vi "Quick Format.vi"(6 "Variant in":variant, 7 "Shift Pressed?":bool, 8 "error in":errorcluster, 10 "QD Combo Box Ref":refnum<vi>, 11 "QD Launch VI Ref":refnum<vi>) -> (0 "error out":errorcluster, 4 "Variant out":variant)   [LabVIEW 2019, in "Quick Format QD.lvlib"]
doc: "Formats selected controls, indicators, and/or constants. The format descriptor must be entered in the Quick Drop window before activating this plugin.\n\nAccepted format descriptors are as follows. The descriptors are not case sensitive.\nDecimal (numeric) - d, dec\nHexadecimal (numeric, string) - h, x, hex\nOctal (numeric) - o, oct\nBinary (numeric) - b, bin\nSI (numeric) - si\nSI notation with specific units (numeric) - freq, sec, volt, amp, ohm, watt\nDecimal notation with specific units (numeric) - db, dbm, dbc\nLocal Time (numeric and timestamp) - time\nUTC Time (numeric and timestamp) - utc\nNormal Display (string) - n, norm\nSlash Codes (string) - \\, slash\nPassword Display (string) - p, pass\nCustom Code (numeric, timestamp) - any valid display format (for example: %f)\n\nAny setting that is applied to a string forces the Display Style to be visible.\nHexadecimal, Octal, and Binary settings applied to numerics forces the radix to be visible.\nHexadecimal, Octal, and Binary settings applied to numerics set the number of displayed digits based on the data type.\nAny elements inside of arrays and clusters are recursively processed.\n\nDefault Shortcut - [5]"
uses:
  Quick Format QD.lvlib
panel:
  # "THE SOFTWARE IS PROVIDED “AS IS” AND THE AUTHOR DISCLAIMS ALL WARRANTIES WITH REGARD TO THIS SOFTWARE INCLUDING ALL IMPLIED WARRANTIES OF MERCHANTABILITY AND FITNESS. IN NO EVENT SHALL THE AUTHOR BE LIABLE FOR ANY SPECIAL, DIRECT, INDIRECT, OR CONSEQUENTIAL DAMAGES OR ANY DAMAGES WHATSOEVER RESULTING FROM LOSS OF USE, DATA OR PROFITS, WHETHER IN AN ACTION OF CONTRACT, NEGLIGENCE OR OTHER TORTIOUS ACTION, ARISING OUT OF OR IN CONNECTION WITH THE USE OR PERFORMANCE OF THIS SOFTWARE."
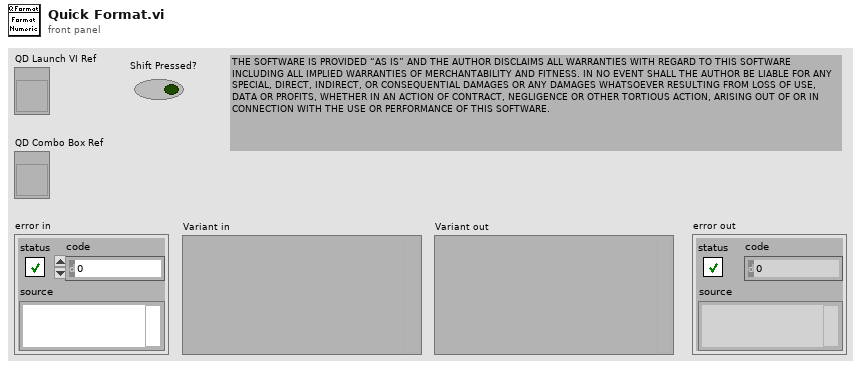
[diagram p1: front panel]
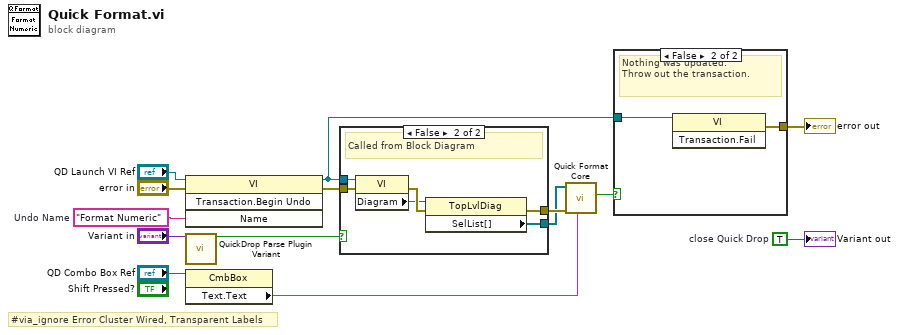
[diagram p0: block diagram]
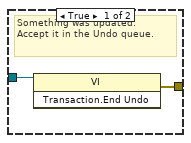
[diagram p2: hidden frame]
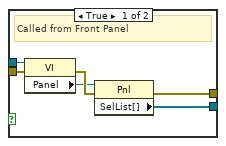
[diagram p3: hidden frame]
diagram:
  w6 = TRUE  # close Quick Drop
  w7 = "Format Numeric"  # Undo Name
  # "#via_ignore Error Cluster Wired, Transparent Labels"
  n1 = invoke on="Invoke Node" class="VI" method="Transaction.Begin Undo"(reference="QD Launch VI Ref", error in="error in", "Name"=w7) -> (reference out=w4:refnum<vi>, error out=w12:errorcluster)  [unwired: 1 in, 2 out]
  n2 = call <vilib>:"QuickDrop Parse Plugin Variant.vi"("QDKS Variant in"="Variant in") -> ("QD Launch VI Panel?"=w5:bool)  [unwired: 12 in, 2 out]
  n3 = property on="Property Node" class="CmbBox"(reference="QD Combo Box Ref") -> ("Text.Text"=w2:string)  [unwired: 1 in, 2 out]
  n4 = case shown="False" w5 {
    tunnel: w12 -> [w20 w26]
    tunnel: w4 -> [w17 w23]
    tunnel: [w15 w21] -> w3
    tunnel: [w18 w24] -> w11
    frame True {
      # "Called from Front Panel"
      n5 = property on="Property Node" class="VI"(reference=w17, error in=w20) -> (error out=w19:errorcluster, "Panel"=w16:refnum<vi>)  [unwired: 1 out]
      n6 = property on="Property Node" class="Pnl"(reference=w16, error in=w19) -> (error out=w18:errorcluster, "SelList[]"=w15:refnum<vi>[])  [unwired: 1 out]
    }
    frame False {
      # "Called from Block Diagram"
      n7 = property on="Property Node" class="VI"(reference=w23, error in=w26) -> (error out=w25:errorcluster, "Diagram"=w22:refnum<vi>)  [unwired: 1 out]
      n8 = property on="Property Node" class="TopLvlDiag"(reference=w22, error in=w25) -> (error out=w24:errorcluster, "SelList[]"=w21:refnum<vi>[])  [unwired: 1 out]
    }
  }
  n9 = call "Quick Format Core.vi"("Format String"=w2, "error in"=w11, "GObjects"=w3) -> ("Successful"=w1:bool)  [unwired: 8 in]
  n10 = case shown="False" w1 {
    tunnel: w4 -> [w27 w29]
    tunnel: [w28 w30] -> w13
    frame True {
      # "Something was updated.\nAccept it in the Undo queue."
      n11 = invoke on="Invoke Node" class="VI" method="Transaction.End Undo"(reference=w27) -> (error out=w28:errorcluster)  [unwired: 2 in, 2 out]
    }
    frame False {
      # "Nothing was updated.\nThrow out the transaction."
      n12 = invoke on="Invoke Node" class="VI" method="Transaction.Fail"(reference=w29) -> (error out=w30:errorcluster)  [unwired: 2 in, 2 out]
    }
  }
  "error out" <- w13
  "Variant out" <- w6
